vi "Target Send Telemetry.vi"(11 "Target Sensors":T1) -> ()   [LabVIEW 2018]
uses:
  Ankle Benchtop Testing Advanced/Target Sensors.ctl
  Ankle Benchtop Testing Advanced/Target Raw Sensors.ctl
  Ankle Benchtop Testing Advanced/Target Filtered Sensors.ctl
  Ankle Benchtop Testing Advanced/Target Telemetry Cluster.ctl
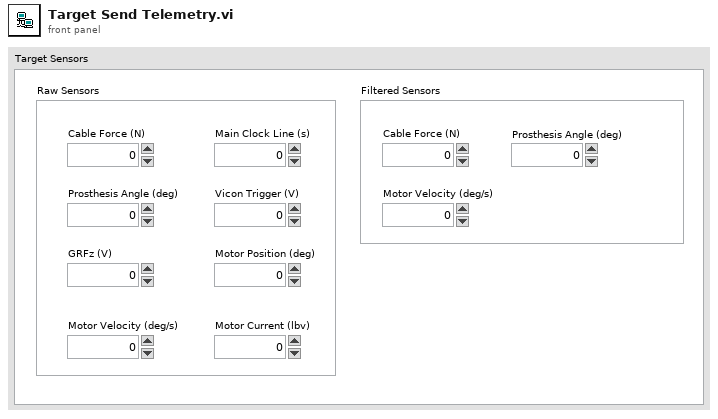
[diagram p1: front panel]
types:
  T1 = typedef "Target Sensors.ctl" = cluster{"Raw Sensors":T2, "Filtered Sensors":T3}
  T2 = typedef "Target Raw Sensors.ctl" = cluster{"Cable Force (N)":dbl, "Prosthesis Angle (deg)":dbl, "Main Clock Line (s)":dbl, "Vicon Trigger (V)":dbl, "GRFz (V)":dbl, "Motor Position (deg)":dbl, "Motor Velocity (deg/s)":dbl, "Motor Current (lbv)":dbl}
  T3 = typedef "Target Filtered Sensors.ctl" = cluster{"Cable Force (N)":dbl, "Prosthesis Angle (deg)":dbl, "Motor Velocity (deg/s)":dbl}
  T4 = typedef "Target Telemetry Cluster.ctl" = cluster{"Target Sensors":T1}
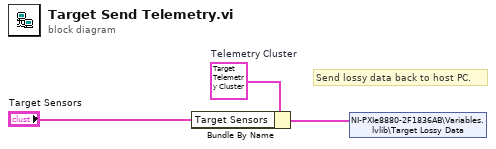
[diagram p0: block diagram]
diagram:
  w3 = T4 {"Target Sensors"={"Raw Sensors"={"Cable Force (N)"=0.0, "Prosthesis Angle (deg)"=0.0, "Main Clock Line (s)"=0.0, "Vicon Trigger (V)"=0.0, "GRFz (V)"=0.0, "Motor Position (deg)"=0.0, "Motor Velocity (deg/s)"=0.0, "Motor Current (lbv)"=0.0}, "Filtered Sensors"={"Cable Force (N)"=0.0, "Prosthesis Angle (deg)"=0.0, "Motor Velocity (deg/s)"=0.0}}}  # Telemetry Cluster
  # "Send lossy data back to host PC."
  n1 = Bundle By Name(cluster=w3, "Target Sensors"="Target Sensors") -> (w2:T4)
  n2 = shared-variable "NI-PXIe8880-2F1836AB\\Variables.lvlib\\Target Lossy Data"(w2) -> ()  [unwired: 1 in, 1 out]
